vi "Driving Simulator.vi"() -> ()   [LabVIEW 2019]
uses:
  <vilib>/Utility/NIReport.llb/Report Type.ctl
  <vilib>/Instr/_visa.llb/VISA Configure Serial Port (Instr).vi
  <vilib>/Utility/inputDevices.llb/joystickAcquire.vi
  <vilib>/addons/_office/excel.llb/Excel Easy Table (num).vi
  <vilib>/Utility/NIReport.llb/NI_report.lvclass
  <vilib>/addons/_office/NI_ReportGenerationToolkit.lvlib
  <vilib>/Utility/NIReport.llb/NI_ReportGenerationCore.lvlib
panel:
  out "BRdisp 3":i32(slide) caption="Brake" scale=0.0..100.0
  out "revStateTest 2":bool caption="Reverse"
  out "hbStateTest 2":bool caption="Hand Brake"
  out "THdisp 2":i32(slide) caption="Throtle" scale=0.0..100.0
  out "SWdisp 2":i32(knob) caption="Steering wheel" scale=0.0..200.0
  out "mPos":cluster{dbl, dbl, dbl}(graph) caption="Motor Positions"
  out "platDisWF":dbl(graph) caption="Displacement"
  out "platPosWF":cluster{"Pitch":dbl, "Roll":dbl, "yaw ":dbl}(graph) caption="Rotations"
  in  "rev":bool caption="reversa"
  in  "hb":bool caption="freno de mano"
  in  "st":i32(knob)=100 caption="volante" scale=0.0..200.0
  in  "br":i32(knob) caption="freno" scale=0.0..100.0
  in  "tr":i32(knob) caption="acelerador" scale=0.0..100.0
  in  "Preferences":bool caption="Edit Simulation Preferences"
  in  "Tab Control 2":enum32{"Input Devices", "IMU", "MCA"}(tab)
  in  "inSel":T1(ring) caption="Select Input Source"
  in  "dispWaveform":bool caption="Display IMU signals?"
  in  "filter":bool=TRUE caption="Filter IMU signals?"
  in  "pitchLIM":dbl=10.0 caption="Pitch Limit"
  in  "xlp":dbl(slide)=0.5 caption="Pitch \nAcceleration \nGain" scale=0.0..0.9 scale format="%#_4g"
  in  "dispMCA":bool caption="Display MCA Output?"
  in  "xhp":dbl(slide)=0.002 caption="Pitch\nVelocity\nGain" scale=0.0..0.02 scale format="%#_4g"
  in  "ylp":dbl(slide)=0.1 caption="Roll\nAcceleration\nGain" scale=0.0..0.2 scale format="%#_4g"
  in  "yhp":dbl(slide)=0.001 caption="Roll\nVelocity\nGain" scale=0.0..0.01 scale format="%#_4g"
  in  "zhp":dbl(slide)=0.02 caption="Heave\nGain" scale=0.0..0.1 scale format="%#_4g"
  in  "rollLIM":dbl=10.0 caption="Roll Limit"
  in  "heaveLIM":dbl=0.01 caption="Heave Limit"
  out "speed":dbl(knob) caption="Speedometer" scale=0.0..100.0
  out "vel":cluster{"vx":dbl, "vy":dbl, "vy":dbl}(graph) caption="Velocity"
  out "acc":cluster{"vx":dbl, "vy":dbl, "vy":dbl}(graph) caption="Acceleration"
  in  "StopSim":bool caption="Stop Simulation"
  out "errorS1":string caption="ERROR Log"
  out "timer":i32(slide) caption="Wating for CARLA to open" scale=0.0..40.0
  in  "sysConf":bool caption="System Configuration"
  in  "Tab Control":T2(tab)
  out "hbStateTest":bool caption="Hand Brake"
  out "revStateTest":bool caption="Reverse"
  out "THdisp":i32(slide) caption="Throtle" scale=0.0..100.0
  in  "startMconf":bool caption="Set Motor Position Manually"
  in  "set":bool caption="Set Current Position as Home"
  in  "m3":i32=90 caption="Motor 3"
  in  "m2":i32=90 caption="Motor 2"
  in  "m1":i32=90 caption="Motor 1"
  in  "extInputsON":bool caption="Imput Devices Connected?"
  in  "controlON":bool caption="Platform Conected?"
  in  "baudRate":i32=115200 caption="Controller Baud Rate"
  in  "XboxON":bool caption="Xbox Controller Connected?"
  in  "TCP Port":i32=10000 caption="CARLA Server TCP Port"
  in  "VISAportC":refnum<visa-resource-name> caption="Controller Serial Port"
  in  "IDbaudRate":i32=115200 caption="Input Devices Baud Rate"
  in  "VISAportID":refnum<visa-resource-name> caption="Input Devices Port"
  out "SWdisp":i32(knob) caption="Steering wheel" scale=0.0..200.0
  out "BRdisp 2":i32(slide) caption="Brake" scale=0.0..100.0
  in  "startIDtest":bool caption="Test Input Devices"
  in  "finishIDtest":bool caption="Finish Testing"
  in  "b":dbl=0.0887 caption="Leg Length"
  in  "a":dbl=0.03 caption="Crank Length"
  in  "z":dbl=0.0887 caption="Platform Height"
  in  "R":dbl=0.0851 caption="Base Radius"
  in  "r":dbl=0.115 caption="Platform Radius"
  in  "record":bool caption="Activate Variable Recording"
  in  "report type":T3=enum."Excel"
  in  "CARLAstat":bool caption="Is CARLA Server Already Running?"
  in  "CARLA Client":path=path "C:/CARLA/PythonAPI/examples/manual_control.py"
  in  "CARLA Server":path=path "C:/CARLA/CarlaUE4.exe"
  in  "Finish":bool caption="Start Simulation"
  out "Status":string caption="Program Status"
  # "* All Dimentions are in meters"
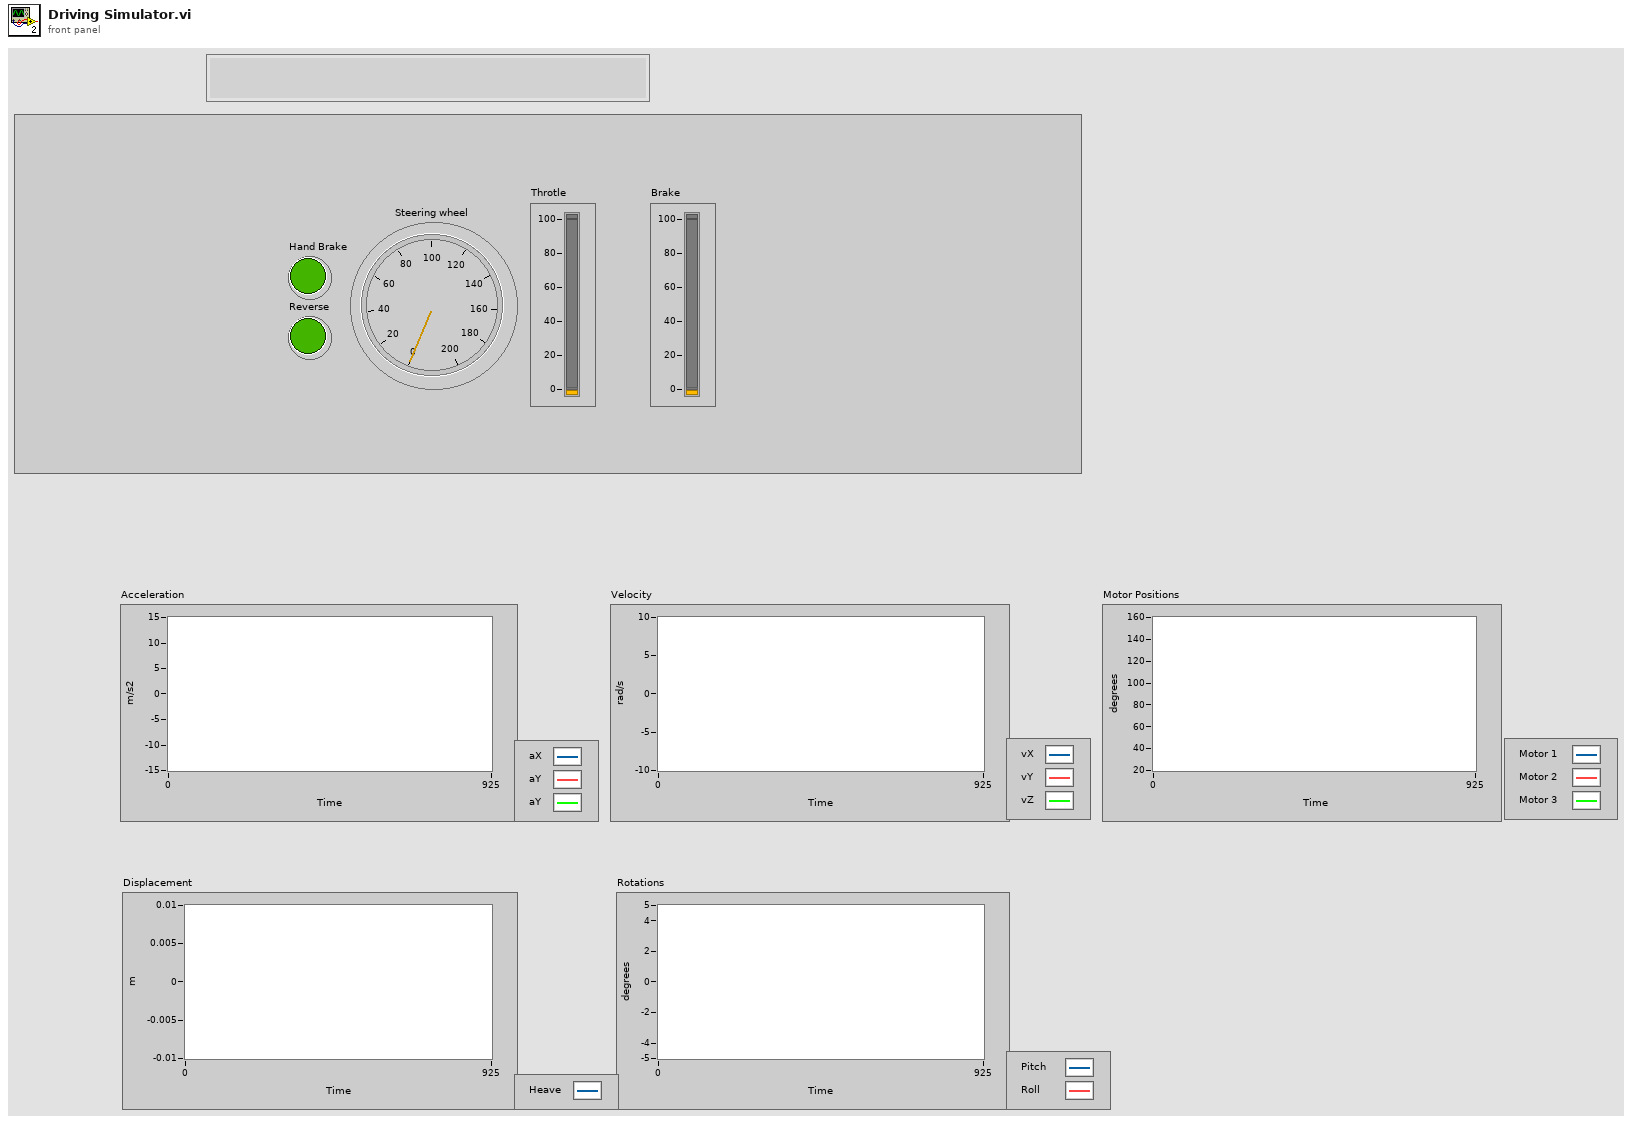
[diagram p1: front panel]
types:
  T1 = enum16{"LabVIEW", "External Devices", "Xbox Controller"}
  T2 = enum32{"Communication", "Platform Dimensions", "Result Recording"}
  T3 = typedef "NI_ReportGenerationCore.lvlib/Report Type.ctl" = enum16{"HTML", "Word", "Excel"}
  T4 = enum8{"Enabled", "Disabled", "Disabled and Grayed Out"}
  T5 = cluster{"st":i32, "tr":i32, "br":i32, "rev":bool, "hb":bool}
  T6 = cluster{"st":i32, "tr":i32, "tr":i32, "hb":bool, "hb":bool}
  T7 = cluster{i32, "Throtle":i32, "Brake":i32, "Reverse":bool, "hand Brake":bool}
  T8 = cluster{"st":i32, "br":i32, "tr":i32, "hb":bool, "rev":bool}
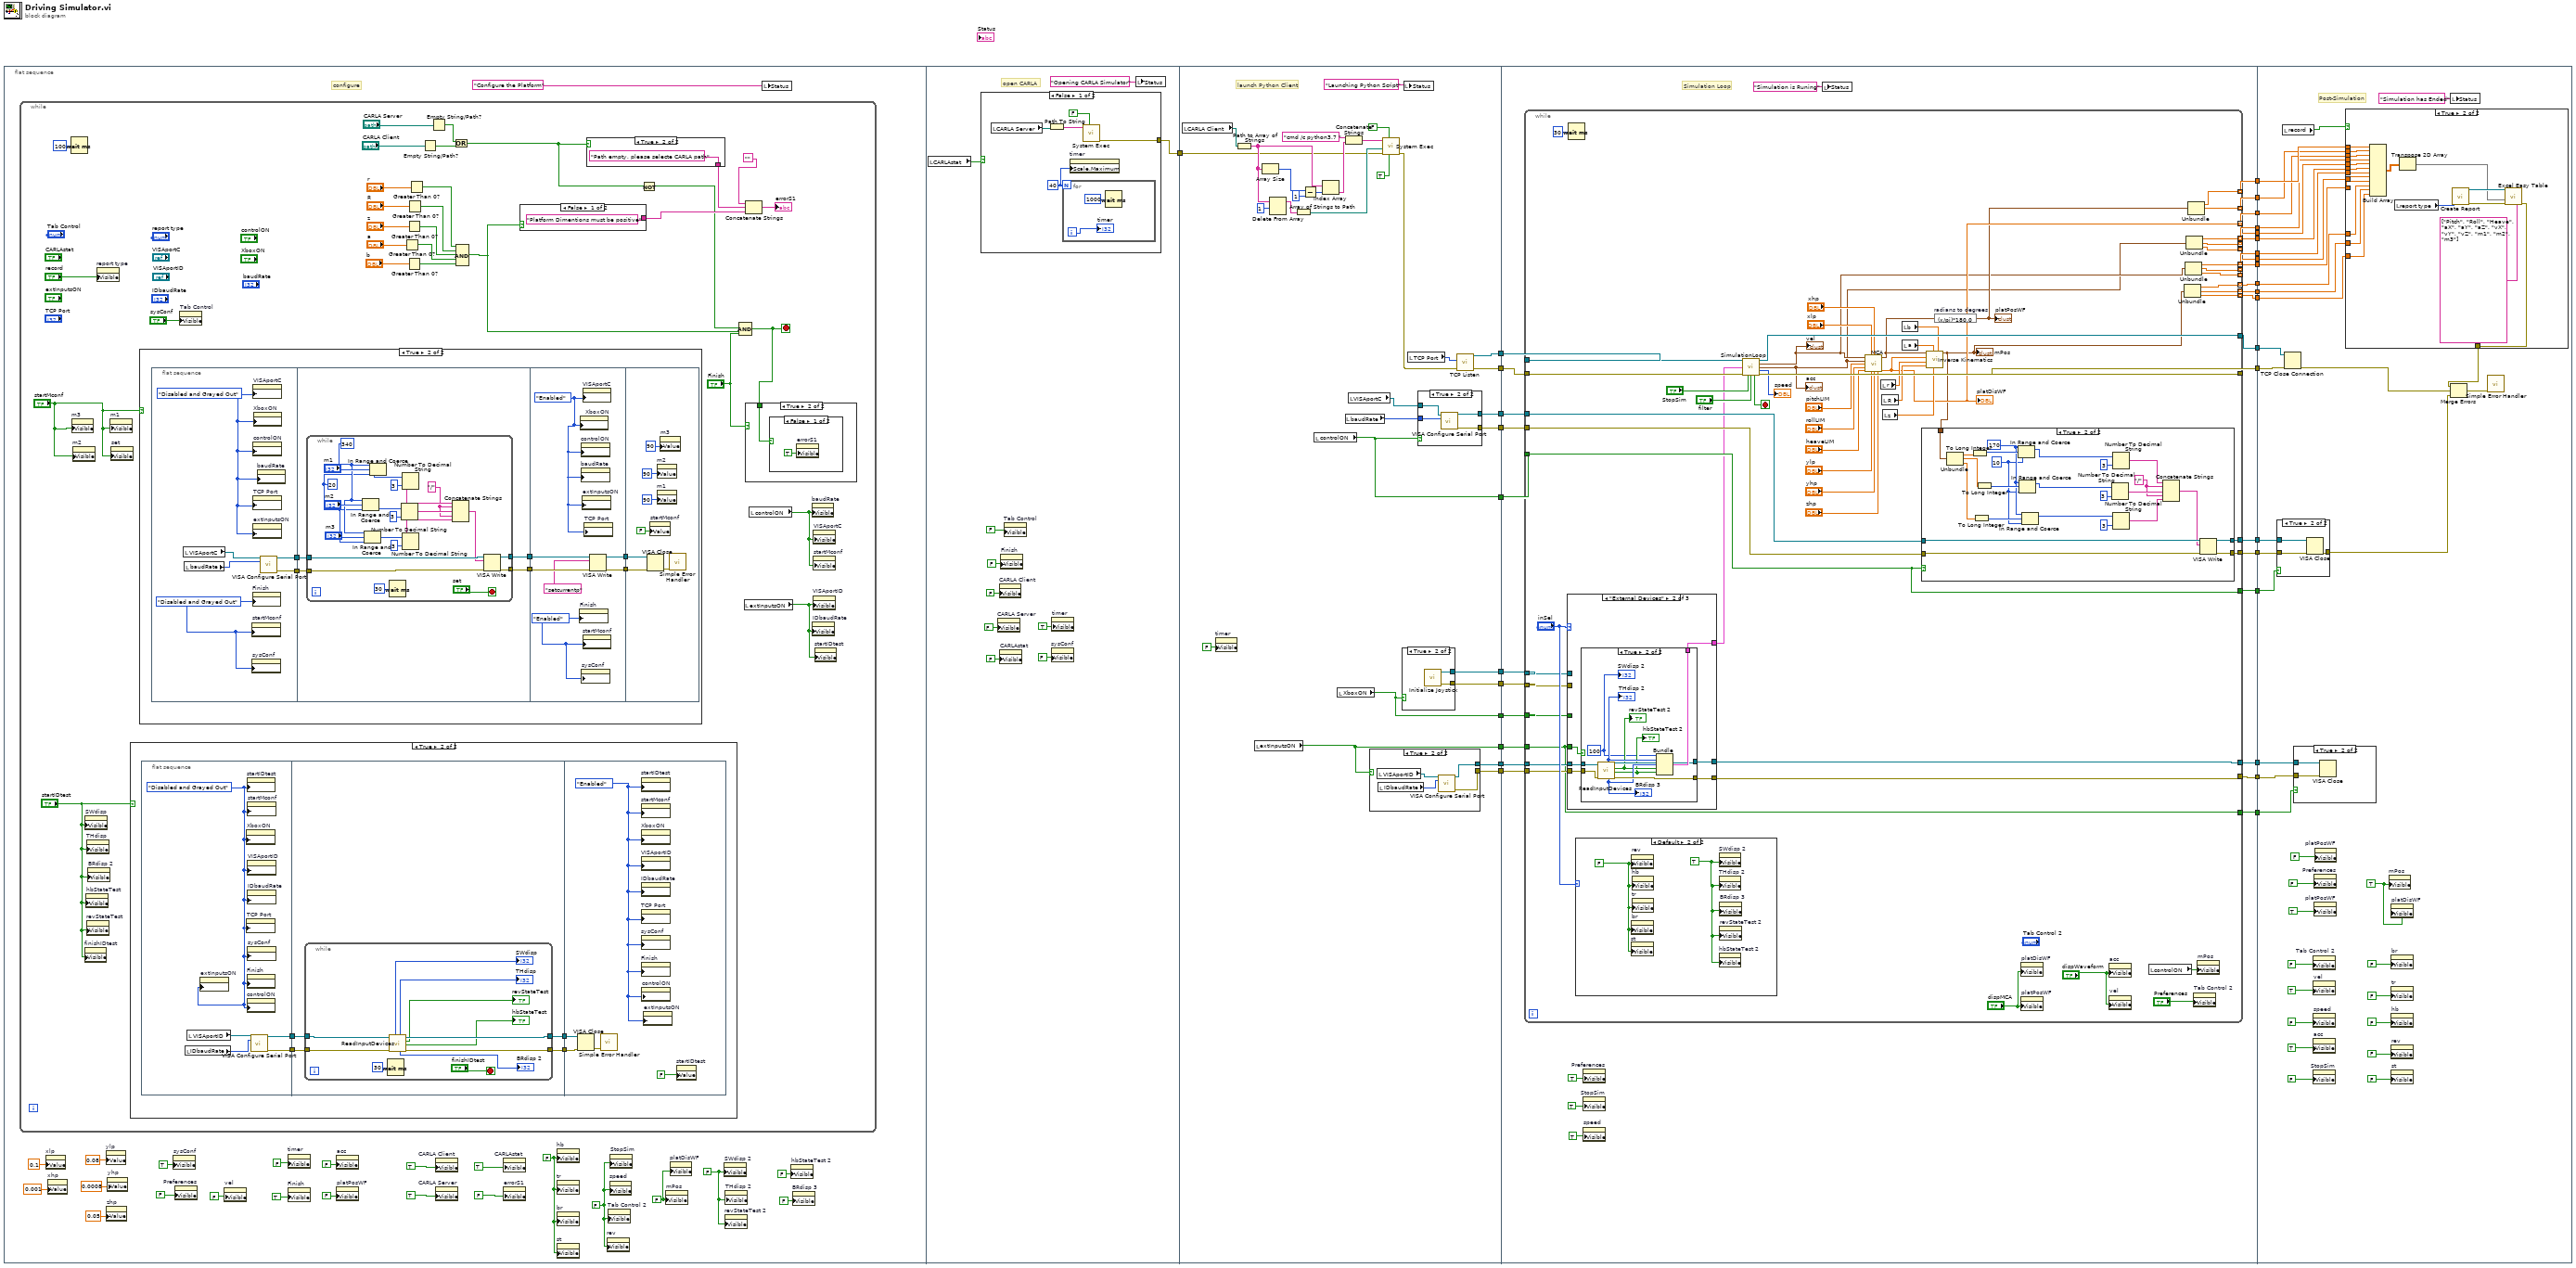
[diagram p0: block diagram]
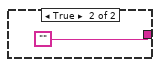
[diagram p4: hidden frame]
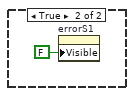
[diagram p6: hidden frame]
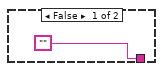
[diagram p7: hidden frame]
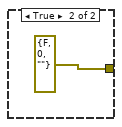
[diagram p8: hidden frame]
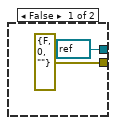
[diagram p9: hidden frame]
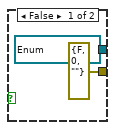
[diagram p10: hidden frame]
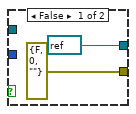
[diagram p11: hidden frame]
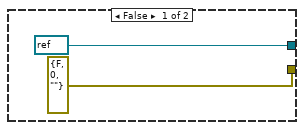
[diagram p12: hidden frame]
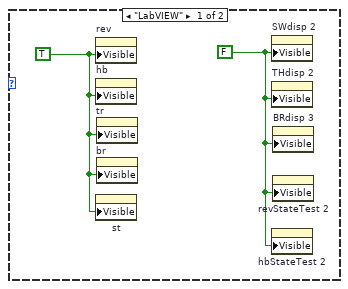
[diagram p13: hidden frame]
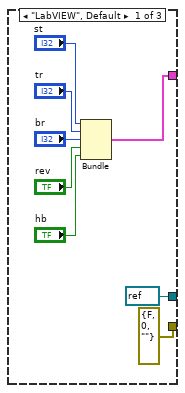
[diagram p14: hidden frame]
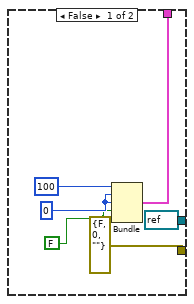
[diagram p15: hidden frame]
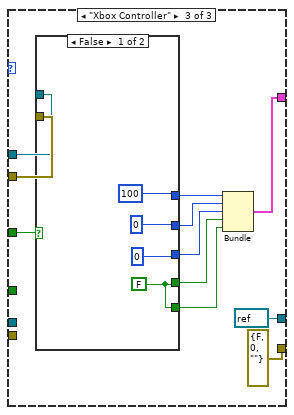
[diagram p16: hidden frame]
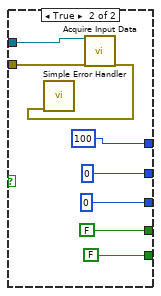
[diagram p17: hidden frame]
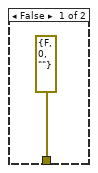
[diagram p19: hidden frame]
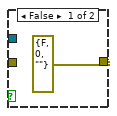
[diagram p20: hidden frame]
diagram:
  n1 = flat-sequence {
    tunnel: [w181] -> w32
    tunnel: w32 -> [w210]
    tunnel: [w208] -> w31
    tunnel: [w207] -> w30
    tunnel: [w205] -> w29
    tunnel: [w204] -> w28
    tunnel: [w199] -> w27
    tunnel: [w202] -> w26
    tunnel: [w201] -> w25
    tunnel: [w200] -> w24
    tunnel: [w194] -> w9
    tunnel: [w193] -> w8
    tunnel: [w192] -> w7
    tunnel: w31 -> [w272]
    tunnel: w30 -> [w271]
    tunnel: [w268] -> w23
    tunnel: [w266] -> w22
    tunnel: w29 -> [w265]
    tunnel: w28 -> [w264]
    tunnel: [w263] -> w21
    tunnel: [w262] -> w20
    tunnel: w27 -> [w261]
    tunnel: [w260] -> w19
    tunnel: w26 -> [w259]
    tunnel: w25 -> [w258]
    tunnel: w24 -> [w257]
    tunnel: [w256] -> w18
    tunnel: [w255] -> w17
    tunnel: [w254] -> w16
    tunnel: [w253] -> w15
    tunnel: [w252] -> w14
    tunnel: [w251] -> w13
    tunnel: [w250] -> w12
    tunnel: [w249] -> w11
    tunnel: [w248] -> w10
    tunnel: w9 -> [w247]
    tunnel: w8 -> [w246]
    tunnel: w7 -> [w245]
    tunnel: [w244] -> w6
    tunnel: [w243] -> w5
    tunnel: [w242] -> w4
    tunnel: [w240] -> w3
    tunnel: [w241] -> w2
    tunnel: [w239] -> w1
    tunnel: w23 -> [w453]
    tunnel: w22 -> [w421]
    tunnel: w21 -> [w439]
    tunnel: w20 -> [w438]
    tunnel: w19 -> [w422]
    tunnel: w18 -> [w436]
    tunnel: w17 -> [w435]
    tunnel: w16 -> [w434]
    tunnel: w15 -> [w433]
    tunnel: w14 -> [w432]
    tunnel: w13 -> [w431]
    tunnel: w12 -> [w430]
    tunnel: w11 -> [w429]
    tunnel: w10 -> [w428]
    tunnel: w6 -> [w420]
    tunnel: w5 -> [w419]
    tunnel: w4 -> [w418]
    tunnel: w3 -> [w416]
    tunnel: w2 -> [w415]
    tunnel: w1 -> [w417]
    frame #0 {
      w35 = FALSE ("Visible")
      w36 = FALSE ("Visible")
      w37 = FALSE ("Visible")
      w38 = FALSE ("Visible")
      # "configure"
      n2 = while {
        stop <- w79 stop-if-true
        n3 = Wait (ms)(milliseconds to wait=u32 100) -> ()  [unwired: 1 out]
        n4 = property on="m3" class="DigNum (strict)"("Visible"="startMconf") -> ()  [unwired: 2 in, 2 out]
        n5 = property on="m2" class="DigNum (strict)"("Visible"="startMconf") -> ()  [unwired: 2 in, 2 out]
        n6 = property on="finishIDtest" class="Bool"("Visible"="startIDtest") -> ()  [unwired: 2 in, 2 out]
        n7 = property on="SWdisp" class="Knob (strict)"("Visible"="startIDtest") -> ()  [unwired: 2 in, 2 out]
        n8 = property on="hbStateTest" class="Bool (strict)"("Visible"="startIDtest") -> ()  [unwired: 2 in, 2 out]
        n9 = property on="THdisp" class="Slide (strict)"("Visible"="startIDtest") -> ()  [unwired: 2 in, 2 out]
        n10 = property on="revStateTest" class="Bool (strict)"("Visible"="startIDtest") -> ()  [unwired: 2 in, 2 out]
        n11 = property on="BRdisp 2" class="Slide (strict)"("Visible"="startIDtest") -> ()  [unwired: 2 in, 2 out]
        n12 = property on="report type" class="Enum (strict)"("Visible"="record") -> ()  [unwired: 2 in, 2 out]
        n13 = property on="m1" class="DigNum (strict)"("Visible"="startMconf") -> ()  [unwired: 2 in, 2 out]
        n14 = property on="set" class="Bool"("Visible"="startMconf") -> ()  [unwired: 2 in, 2 out]
        n15 = case shown="True" "startIDtest" {
          frame False {
          }
          frame True {
            n16 = flat-sequence {
              tunnel: [w94] -> w89
              tunnel: [w93] -> w88
              tunnel: w89 -> [w97]
              tunnel: w88 -> [w98]
              tunnel: [w96] -> w87
              tunnel: [w95] -> w86
              tunnel: w87 -> [w112]
              tunnel: w86 -> [w111]
              frame #0 {
                w90 = T4."Disabled and Grayed Out" ("Disabled")
                n17 = local read "IDbaudRate"() -> (w91:i32)
                n18 = local read "VISAportID"() -> (w92:refnum<visa-resource-name>)
                n19 = property on="extInputsON" class="Bool (strict)"("DisabledEnum"=w90) -> ()  [unwired: 2 in, 2 out]
                n20 = property on="XboxON" class="Bool (strict)"("DisabledEnum"=w90) -> ()  [unwired: 2 in, 2 out]
                n21 = property on="TCP Port" class="DigNum (strict)"("DisabledEnum"=w90) -> ()  [unwired: 2 in, 2 out]
                n22 = property on="startIDtest" class="Bool (strict)"("DisabledEnum"=w90) -> ()  [unwired: 2 in, 2 out]
                n23 = property on="Finish" class="Bool"("DisabledEnum"=w90) -> ()  [unwired: 2 in, 2 out]
                n24 = property on="controlON" class="Bool (strict)"("DisabledEnum"=w90) -> ()  [unwired: 2 in, 2 out]
                n25 = property on="startMconf" class="Bool (strict)"("DisabledEnum"=w90) -> ()  [unwired: 2 in, 2 out]
                n26 = property on="VISAportID" class="VISAName"("DisabledEnum"=w90) -> ()  [unwired: 2 in, 2 out]
                n27 = property on="IDbaudRate" class="DigNum (strict)"("DisabledEnum"=w90) -> ()  [unwired: 2 in, 2 out]
                n28 = property on="sysConf" class="Bool (strict)"("DisabledEnum"=w90) -> ()  [unwired: 2 in, 2 out]
                n29 = call-poly "VISA Configure Serial Port"("VISA resource name"=w92, "baud rate (9600)"=w91) -> ("VISA resource name out"=w94:refnum<visa-resource-name>, "error out"=w93:errorcluster)  [unwired: 12 in]
              }
              frame #1 {
                n30 = while {
                  tunnel: w98 -> [w106]
                  tunnel: w97 -> [w107]
                  tunnel: [w105] -> w96
                  tunnel: [w104] -> w95
                  stop <- "finishIDtest" stop-if-true
                  n31 = Wait (ms)(milliseconds to wait=u32 30) -> ()  [unwired: 1 out]
                  n32 = call "ReadInputDevices.vi"("error in (no error)"=w106, "VISA Refnum in"=w107) -> ("error out"=w104:errorcluster, "hand Brake"=→"hbStateTest":bool, "Reverse"=→"revStateTest":bool, "VISA Refnum out"=w105:refnum<visa-resource-name>, "Brake"=→"BRdisp 2":i32, "Throtle"=→"THdisp":i32, "Steering Wheel"=→"SWdisp":i32)  [unwired: 3 in]
                }
              }
              frame #2 {
                w110 = T4."Enabled" ("Disabled")
                n33 = VISA Close(VISA resource name=w112, error in (no error)=w111) -> (error out=w114:errorcluster)
                n34 = call <vilib>:"Simple Error Handler.vi"("error in (no error)"=w114) -> ()  [unwired: 4 in, 5 out]
                n35 = property on="startIDtest" class="Bool (strict)"("DisabledEnum"=w110) -> ()  [unwired: 2 in, 2 out]
                n36 = property on="startMconf" class="Bool (strict)"("DisabledEnum"=w110) -> ()  [unwired: 2 in, 2 out]
                n37 = property on="XboxON" class="Bool (strict)"("DisabledEnum"=w110) -> ()  [unwired: 2 in, 2 out]
                n38 = property on="VISAportID" class="VISAName"("DisabledEnum"=w110) -> ()  [unwired: 2 in, 2 out]
                n39 = property on="IDbaudRate" class="DigNum (strict)"("DisabledEnum"=w110) -> ()  [unwired: 2 in, 2 out]
                n40 = property on="TCP Port" class="DigNum (strict)"("DisabledEnum"=w110) -> ()  [unwired: 2 in, 2 out]
                n41 = property on="sysConf" class="Bool (strict)"("DisabledEnum"=w110) -> ()  [unwired: 2 in, 2 out]
                n42 = property on="Finish" class="Bool"("DisabledEnum"=w110) -> ()  [unwired: 2 in, 2 out]
                n43 = property on="controlON" class="Bool (strict)"("DisabledEnum"=w110) -> ()  [unwired: 2 in, 2 out]
                n44 = property on="extInputsON" class="Bool (strict)"("DisabledEnum"=w110) -> ()  [unwired: 2 in, 2 out]
                n45 = property on="startIDtest" class="Bool (strict)"("Value"=FALSE ("startMconf")) -> ()  [unwired: 2 in, 2 out]
              }
            }
          }
        }
        n46 = case shown="True" "startMconf" {
          frame False {
          }
          frame True {
            n47 = flat-sequence {
              tunnel: [w124] -> w120
              tunnel: [w123] -> w119
              tunnel: w120 -> [w129]
              tunnel: w119 -> [w130]
              tunnel: [w128] -> w118
              tunnel: [w127] -> w117
              tunnel: w118 -> [w159]
              tunnel: w117 -> [w158]
              tunnel: [w156] -> w116
              tunnel: [w155] -> w115
              tunnel: w116 -> [w166]
              tunnel: w115 -> [w165]
              frame #0 {
                w122 = T4."Disabled and Grayed Out" ("Disabled")
                w121 = T4."Disabled and Grayed Out" ("Disabled")
                n48 = local read "VISAportC"() -> (w126:refnum<visa-resource-name>)
                n49 = local read "baudRate"() -> (w125:i32)
                n50 = property on="startMconf" class="Bool (strict)"("DisabledEnum"=w122) -> ()  [unwired: 2 in, 2 out]
                n51 = property on="sysConf" class="Bool (strict)"("DisabledEnum"=w122) -> ()  [unwired: 2 in, 2 out]
                n52 = property on="Finish" class="Bool"("DisabledEnum"=w122) -> ()  [unwired: 2 in, 2 out]
                n53 = property on="VISAportC" class="VISAName"("DisabledEnum"=w121) -> ()  [unwired: 2 in, 2 out]
                n54 = property on="controlON" class="Bool (strict)"("DisabledEnum"=w121) -> ()  [unwired: 2 in, 2 out]
                n55 = property on="TCP Port" class="DigNum (strict)"("DisabledEnum"=w121) -> ()  [unwired: 2 in, 2 out]
                n56 = property on="extInputsON" class="Bool (strict)"("DisabledEnum"=w121) -> ()  [unwired: 2 in, 2 out]
                n57 = property on="XboxON" class="Bool (strict)"("DisabledEnum"=w121) -> ()  [unwired: 2 in, 2 out]
                n58 = property on="baudRate" class="DigNum (strict)"("DisabledEnum"=w121) -> ()  [unwired: 2 in, 2 out]
                n59 = call-poly "VISA Configure Serial Port"("VISA resource name"=w126, "baud rate (9600)"=w125) -> ("VISA resource name out"=w124:refnum<visa-resource-name>, "error out"=w123:errorcluster)  [unwired: 12 in]
              }
              frame #1 {
                n60 = while {
                  tunnel: w130 -> [w152]
                  tunnel: w129 -> [w151]
                  tunnel: [w134] -> w128
                  tunnel: [w133] -> w127
                  stop <- "set" stop-if-true
                  w135 = 20 ("lower limit")
                  w136 = 340 ("upper limit")
                  w144 = "/"
                  n61 = In Range and Coerce(upper limit=w136, x="m2", lower limit=w135) -> (coerced(x)=w138:i32)  [unwired: 1 out]
                  n62 = In Range and Coerce(upper limit=w136, x="m3", lower limit=w135) -> (coerced(x)=w137:i32)  [unwired: 1 out]
                  n63 = In Range and Coerce(upper limit=w136, x="m1", lower limit=w135) -> (coerced(x)=w141:i32)  [unwired: 1 out]
                  n64 = Wait (ms)(milliseconds to wait=u32 30) -> ()  [unwired: 1 out]
                  n65 = Number To Decimal String(number=w138, width (-)=i16 3) -> (decimal integer string=w149:string)
                  n66 = Number To Decimal String(number=w141, width (-)=i16 3) -> (decimal integer string=w148:string)
                  n67 = Number To Decimal String(number=w137, width (-)=i16 3) -> (decimal integer string=w150:string)
                  n68 = Concatenate Strings(w148, w144, w149, w144, w150) -> (w143:string)
                  n69 = VISA Write(VISA resource name=w151, write buffer=w143, error in (no error)=w152) -> (VISA resource name out=w134:refnum<visa-resource-name>, error out=w133:errorcluster)  [unwired: 1 out]
                }
              }
              frame #2 {
                w153 = T4."Enabled" ("Disabled")
                w154 = T4."Enabled" ("Disabled")
                n70 = property on="Finish" class="Bool"("DisabledEnum"=w153) -> ()  [unwired: 2 in, 2 out]
                n71 = property on="XboxON" class="Bool (strict)"("DisabledEnum"=w154) -> ()  [unwired: 2 in, 2 out]
                n72 = property on="controlON" class="Bool (strict)"("DisabledEnum"=w154) -> ()  [unwired: 2 in, 2 out]
                n73 = property on="baudRate" class="DigNum (strict)"("DisabledEnum"=w154) -> ()  [unwired: 2 in, 2 out]
                n74 = property on="sysConf" class="Bool (strict)"("DisabledEnum"=w153) -> ()  [unwired: 2 in, 2 out]
                n75 = property on="extInputsON" class="Bool (strict)"("DisabledEnum"=w154) -> ()  [unwired: 2 in, 2 out]
                n76 = property on="VISAportC" class="VISAName"("DisabledEnum"=w154) -> ()  [unwired: 2 in, 2 out]
                n77 = property on="startMconf" class="Bool (strict)"("DisabledEnum"=w153) -> ()  [unwired: 2 in, 2 out]
                n78 = property on="TCP Port" class="DigNum (strict)"("DisabledEnum"=w154) -> ()  [unwired: 2 in, 2 out]
                n79 = VISA Write(VISA resource name=w159, write buffer="setcurrentp", error in (no error)=w158) -> (VISA resource name out=w156:refnum<visa-resource-name>, error out=w155:errorcluster)  [unwired: 1 out]
              }
              frame #3 {
                n80 = VISA Close(VISA resource name=w166, error in (no error)=w165) -> (error out=w164:errorcluster)
                n81 = property on="startMconf" class="Bool (strict)"("Value"=FALSE ("startMconf")) -> ()  [unwired: 2 in, 2 out]
                n82 = property on="m2" class="DigNum (strict)"("Value"=90 ("m2")) -> ()  [unwired: 2 in, 2 out]
                n83 = property on="m1" class="DigNum (strict)"("Value"=90 ("m1")) -> ()  [unwired: 2 in, 2 out]
                n84 = property on="m3" class="DigNum (strict)"("Value"=90 ("m3")) -> ()  [unwired: 2 in, 2 out]
                n85 = call <vilib>:"Simple Error Handler.vi"("error in (no error)"=w164) -> ()  [unwired: 4 in, 5 out]
              }
            }
          }
        }
        n86 = property on="Tab Control" class="TabCtl (strict)"("Visible"="sysConf") -> ()  [unwired: 2 in, 2 out]
        n87 = Greater Than 0?(x="a") -> (x > 0?=w73:bool)
        n88 = Greater Than 0?(x="z") -> (x > 0?=w74:bool)
        n89 = Greater Than 0?(x="b") -> (x > 0?=w72:bool)
        n90 = Greater Than 0?(x="R") -> (x > 0?=w75:bool)
        n91 = Greater Than 0?(x="r") -> (x > 0?=w76:bool)
        n92 = Empty String/Path?(string/path="CARLA Client") -> (empty?=w78:bool)
        n93 = Empty String/Path?(string/path="CARLA Server") -> (empty?=w83:bool)
        n94 = Or(x=w83, y=w78) -> (x .or. y?=w68:bool)
        n95 = Compound Arithmetic op=AND(w76, w75, w74, w73, w72) -> (w69:bool)
        n96 = case shown="False" w69 {
          tunnel: ["Platform Dimentions must be positive" ""] -> w71
          frame False {
          }
          frame True {
          }
        }
        n97 = case shown="True" w68 {
          tunnel: ["" "Path empty, please selecte CARLA path" ("string")] -> w81
          frame False {
          }
          frame True {
          }
        }
        n98 = Not(x=w68) -> (.not. x?=w67:bool)
        n99 = Compound Arithmetic op=AND(w67, w69, "Finish") -> (w79:bool)
        n100 = local read "extInputsON"() -> (w56:bool)
        n101 = Concatenate Strings("", w81, w71) -> (→"errorS1":string)
        n102 = case shown="True" "Finish" {
          tunnel: w79 -> [_ w169]
          frame False {
          }
          frame True {
            n103 = case shown="False" w169 {
              frame False {
                n104 = property on="errorS1" class="Str"("Visible"=TRUE) -> ()  [unwired: 2 in, 2 out]
              }
              frame True {
                n105 = property on="errorS1" class="Str"("Visible"=FALSE) -> ()  [unwired: 2 in, 2 out]
              }
            }
          }
        }
        n106 = local read "controlON"() -> (w59:bool)
        n107 = property on="baudRate" class="DigNum (strict)"("Visible"=w59) -> ()  [unwired: 2 in, 2 out]
        n108 = property on="IDbaudRate" class="DigNum (strict)"("Visible"=w56) -> ()  [unwired: 2 in, 2 out]
        n109 = property on="VISAportID" class="VISAName"("Visible"=w56) -> ()  [unwired: 2 in, 2 out]
        n110 = property on="VISAportC" class="VISAName"("Visible"=w59) -> ()  [unwired: 2 in, 2 out]
        n111 = property on="startMconf" class="Bool (strict)"("Visible"=w59) -> ()  [unwired: 2 in, 2 out]
        n112 = property on="startIDtest" class="Bool (strict)"("Visible"=w56) -> ()  [unwired: 2 in, 2 out]
      }
      n113 = property on="xlp" class="Slide (strict)"("Value"=0.1 ("xlp")) -> ()  [unwired: 2 in, 2 out]
      n114 = property on="xhp" class="Slide (strict)"("Value"=0.001 ("xhp")) -> ()  [unwired: 2 in, 2 out]
      n115 = property on="ylp" class="Slide (strict)"("Value"=0.08 ("ylp")) -> ()  [unwired: 2 in, 2 out]
      n116 = property on="zhp" class="Slide (strict)"("Value"=0.05 ("zhp")) -> ()  [unwired: 2 in, 2 out]
      n117 = property on="yhp" class="Slide (strict)"("Value"=0.0008 ("yhp")) -> ()  [unwired: 2 in, 2 out]
      n118 = property on="sysConf" class="Bool (strict)"("Visible"=TRUE) -> ()  [unwired: 2 in, 2 out]
      n119 = property on="Preferences" class="Bool (strict)"("Visible"=FALSE) -> ()  [unwired: 2 in, 2 out]
      n120 = property on="vel" class="WFChart (strict)"("Visible"=FALSE) -> ()  [unwired: 2 in, 2 out]
      n121 = property on="timer" class="Slide (strict)"("Visible"=FALSE) -> ()  [unwired: 2 in, 2 out]
      n122 = property on="Finish" class="Bool"("Visible"=TRUE) -> ()  [unwired: 2 in, 2 out]
      n123 = property on="acc" class="WFChart (strict)"("Visible"=FALSE) -> ()  [unwired: 2 in, 2 out]
      n124 = property on="platPosWF" class="WFChart (strict)"("Visible"=FALSE) -> ()  [unwired: 2 in, 2 out]
      n125 = property on="CARLA Client" class="Path"("Visible"=TRUE) -> ()  [unwired: 2 in, 2 out]
      n126 = property on="CARLA Server" class="Path"("Visible"=TRUE) -> ()  [unwired: 2 in, 2 out]
      n127 = property on="CARLAstat" class="Bool (strict)"("Visible"=TRUE) -> ()  [unwired: 2 in, 2 out]
      n128 = property on="errorS1" class="Str"("Visible"=FALSE) -> ()  [unwired: 2 in, 2 out]
      n129 = property on="hb" class="Bool (strict)"("Visible"=w38) -> ()  [unwired: 2 in, 2 out]
      n130 = property on="tr" class="Knob (strict)"("Visible"=w38) -> ()  [unwired: 2 in, 2 out]
      n131 = property on="br" class="Knob (strict)"("Visible"=w38) -> ()  [unwired: 2 in, 2 out]
      n132 = property on="st" class="Knob (strict)"("Visible"=w38) -> ()  [unwired: 2 in, 2 out]
      n133 = property on="rev" class="Bool (strict)"("Visible"=w37) -> ()  [unwired: 2 in, 2 out]
      n134 = property on="Tab Control 2" class="TabCtl (strict)"("Visible"=w37) -> ()  [unwired: 2 in, 2 out]
      n135 = property on="speed" class="Knob (strict)"("Visible"=w37) -> ()  [unwired: 2 in, 2 out]
      n136 = property on="StopSim" class="Bool"("Visible"=w37) -> ()  [unwired: 2 in, 2 out]
      n137 = property on="mPos" class="WFChart (strict)"("Visible"=w36) -> ()  [unwired: 2 in, 2 out]
      n138 = property on="platDisWF" class="WFChart (strict)"("Visible"=w36) -> ()  [unwired: 2 in, 2 out]
      n139 = property on="SWdisp 2" class="Knob (strict)"("Visible"=w35) -> ()  [unwired: 2 in, 2 out]
      n140 = property on="revStateTest 2" class="Bool (strict)"("Visible"=w35) -> ()  [unwired: 2 in, 2 out]
      n141 = property on="THdisp 2" class="Slide (strict)"("Visible"=w35) -> ()  [unwired: 2 in, 2 out]
      n142 = local write "Status"("Configure the Platform" ("String")) -> ()
      n143 = property on="hbStateTest 2" class="Bool (strict)"("Visible"=FALSE) -> ()  [unwired: 2 in, 2 out]
      n144 = property on="BRdisp 3" class="Slide (strict)"("Visible"=FALSE) -> ()  [unwired: 2 in, 2 out]
    }
    frame #1 {
      # "open CARLA"
      n145 = local read "CARLAstat"() -> (w174:bool)
      n146 = case shown="False" w174 {
        tunnel: [w186 errorcluster {"status"=FALSE, "code"=0, "source"=""} ("error out")] -> w181
        frame False {
          w185 = 40
          n147 = local read "CARLA Server"() -> (w184:path)
          n148 = Path To String(path=w184) -> (string=w188:string)
          n149 = for {
            N: w185 -> [_]
            i -> [w190]
            n150 = Wait (ms)(milliseconds to wait=u32 1000) -> ()  [unwired: 1 out]
            "timer" <- w190
          }
          n151 = property on="timer" class="Slide (strict)"("Scale.Maximum"=w185) -> ()  [unwired: 2 in, 2 out]
          n152 = call <vilib>:"System Exec.vi"("wait until completion? (T)"=FALSE, "command line"=w188) -> ("error out"=w186:errorcluster)  [unwired: 6 in, 3 out]
        }
        frame True {
        }
      }
      n153 = property on="CARLA Server" class="Path"("Visible"=FALSE) -> ()  [unwired: 2 in, 2 out]
      n154 = property on="CARLA Client" class="Path"("Visible"=FALSE) -> ()  [unwired: 2 in, 2 out]
      n155 = property on="CARLAstat" class="Bool (strict)"("Visible"=FALSE) -> ()  [unwired: 2 in, 2 out]
      n156 = property on="Finish" class="Bool"("Visible"=FALSE) -> ()  [unwired: 2 in, 2 out]
      n157 = property on="Tab Control" class="TabCtl (strict)"("Visible"=FALSE) -> ()  [unwired: 2 in, 2 out]
      n158 = property on="sysConf" class="Bool (strict)"("Visible"=FALSE) -> ()  [unwired: 2 in, 2 out]
      n159 = property on="timer" class="Slide (strict)"("Visible"=TRUE) -> ()  [unwired: 2 in, 2 out]
      n160 = local write "Status"("Opening CARLA Simulator" ("String")) -> ()
    }
    frame #2 {
      # "launch Python Client"
      n161 = local read "CARLA Client"() -> (w196:path)
      n162 = property on="timer" class="Slide (strict)"("Visible"=FALSE) -> ()  [unwired: 2 in, 2 out]
      n163 = Path to Array of Strings(0:w196) -> (2:w216:string[])  [unwired: 1 out]
      n164 = local read "extInputsON"() -> (w192:bool)
      n165 = Array Size(array=w216) -> (size(s)=w215:i32)
      n166 = Delete From Array(array=w216, length=1) -> (array with subset deleted=w218:string[])  [unwired: 1 in, 1 out]
      n167 = Array of Strings to Path(0:w218) -> (2:w221:path)  [unwired: 1 in]
      n168 = Subtract(x=w215, y=1) -> (x-y=w217:i32)
      n169 = local read "controlON"() -> (w199:bool)
      n170 = Index Array(array=w216, index=w217) -> (element=w220:string)
      n171 = local read "XboxON"() -> (w200:bool)
      n172 = local read "baudRate"() -> (w198:i32)
      n173 = Concatenate Strings("cmd /c python3.7 " ("string"), w220) -> (w219:string)
      n174 = local read "VISAportC"() -> (w195:refnum<visa-resource-name>)
      n175 = case shown="True" w192 {
        tunnel: [refnum<visa-resource-name> refnum ("VISA resource name out") w228] -> w194
        tunnel: [errorcluster {"status"=FALSE, "code"=0, "source"=""} ("error out") w227] -> w193
        frame False {
        }
        frame True {
          n176 = local read "VISAportID"() -> (w225:refnum<visa-resource-name>)
          n177 = local read "IDbaudRate"() -> (w226:i32)
          n178 = call-poly "VISA Configure Serial Port"("VISA resource name"=w225, "baud rate (9600)"=w226) -> ("VISA resource name out"=w228:refnum<visa-resource-name>, "error out"=w227:errorcluster)  [unwired: 12 in]
        }
      }
      n179 = call <vilib>:"System Exec.vi"("run minimized? (F)"=TRUE, "wait until completion? (T)"=FALSE, "error in (no error)"=w210, "working directory"=w221, "command line"=w219) -> ("error out"=w203:errorcluster)  [unwired: 3 in, 3 out]
      n180 = case shown="True" w200 {
        tunnel: [w230 w232] -> w202
        tunnel: [errorcluster {"status"=FALSE, "code"=0, "source"=""} ("error out") w231] -> w201
        frame False {
          w230 = refnum<k1> refnum items=["JOYSTICK"] ("device ID")
        }
        frame True {
          n181 = call <vilib>:"Initialize Joystick.vi"() -> ("error out"=w231:errorcluster, "device ID"=w232:refnum<k1>)  [unwired: 10 in]
        }
      }
      n182 = local write "Status"("Launching Python Script" ("String")) -> ()
      n183 = local read "TCP Port"() -> (w197:i32)
      n184 = case shown="True" w199 {
        tunnel: w198 -> [_ w238]
        tunnel: [refnum<visa-resource-name> refnum ("VISA resource name out") w237] -> w205
        tunnel: [errorcluster {"status"=FALSE, "code"=0, "source"=""} ("error out") w236] -> w204
        tunnel: w195 -> [_ w235]
        frame False {
        }
        frame True {
          n185 = call-poly "VISA Configure Serial Port"("VISA resource name"=w235, "baud rate (9600)"=w238) -> ("VISA resource name out"=w237:refnum<visa-resource-name>, "error out"=w236:errorcluster)  [unwired: 12 in]
        }
      }
      n186 = call <vilib>:"TCP Listen.vi"("error in (no error)"=w203, "port"=w197) -> ("error out"=w207:errorcluster, "connection ID"=w208:refnum<k5>)  [unwired: 5 in, 3 out]
    }
    frame #3 {
      # "Simulation Loop"
      n187 = while {
        tunnel: w272 -> [w331]
        tunnel: [w329] -> w266
        tunnel: w271 -> [w330]
        tunnel: [w328] -> w268
        tunnel: w265 -> [w311]
        tunnel: w264 -> [w312]
        tunnel: [w310] -> w263
        tunnel: [w309] -> w262
        tunnel: w261 -> [w308]
        tunnel: [w308] -> w260
        tunnel: w259 -> [w307]
        tunnel: w258 -> [w306]
        tunnel: w257 -> [w305]
        tunnel: [w296] -> w256 mode=indexing
        tunnel: [w295] -> w255 mode=indexing
        tunnel: [w293] -> w254 mode=indexing
        tunnel: [w292] -> w253 mode=indexing
        tunnel: [w291] -> w252 mode=indexing
        tunnel: [w290] -> w251 mode=indexing
        tunnel: [w289] -> w250 mode=indexing
        tunnel: [w288] -> w249 mode=indexing
        tunnel: [w287] -> w248 mode=indexing
        tunnel: w247 -> [w282]
        tunnel: w246 -> [w281]
        tunnel: w245 -> [w278]
        tunnel: [w280] -> w244
        tunnel: [w279] -> w243
        tunnel: [w278] -> w242
        tunnel: [w276] -> w239 mode=indexing
        tunnel: [w275] -> w240 mode=indexing
        tunnel: [w274] -> w241 mode=indexing
        stop <- w327 stop-if-true
        n188 = case shown="\"External Devices\"" "inSel" {
          tunnel: w307 -> [_ _ w400]
          tunnel: w306 -> [_ _ w401]
          tunnel: w305 -> [_ _ w402]
          tunnel: [w364 w375 w394] -> w283
          tunnel: w282 -> [_ w374 _]
          tunnel: w281 -> [_ w373 _]
          tunnel: w278 -> [_ w372 _]
          tunnel: [refnum<visa-resource-name> refnum ("VISA Refnum out") w371 refnum<visa-resource-name> refnum ("VISA Refnum out")] -> w280
          tunnel: [errorcluster {"status"=FALSE, "code"=0, "source"=""} ("error out") w370 errorcluster {"status"=FALSE, "code"=0, "source"=""} ("error out")] -> w279
          frame "LabVIEW", Default {
            n189 = Bundle("st"="st", "tr"="tr", "br"="br", "rev"="rev", "hb"="hb") -> (w364:T5)  [unwired: 1 in]
          }
          frame "External Devices" {
            n190 = case shown="True" w372 {
              tunnel: [w378 w391] -> w375
              tunnel: w374 -> [_ w390]
              tunnel: w373 -> [_ w389]
              tunnel: [refnum<visa-resource-name> refnum ("VISA Refnum out") w388] -> w371
              tunnel: [errorcluster {"status"=FALSE, "code"=0, "source"=""} ("error out") w387] -> w370
              frame False {
                w379 = FALSE ("hb")
                w380 = 0 ("tr")
                n191 = Bundle("st"=100, "tr"=w380, "tr"=w380, "hb"=w379, "hb"=w379) -> (w378:T6)  [unwired: 1 in]
              }
              frame True {
                w382 = 100
                n192 = call "ReadInputDevices.vi"("error in (no error)"=w389, "VISA Refnum in"=w390) -> ("error out"=w387:errorcluster, "hand Brake"=w383:bool, "Reverse"=w384:bool, "VISA Refnum out"=w388:refnum<visa-resource-name>, "Brake"=w385:i32, "Throtle"=w386:i32)  [unwired: 3 in, 1 out]
                "THdisp 2" <- w386
                "BRdisp 3" <- w385
                "revStateTest 2" <- w384
                "hbStateTest 2" <- w383
                n193 = Bundle(w382, "Throtle"=w386, "Brake"=w385, "Reverse"=w384, "hand Brake"=w383) -> (w391:T7)  [unwired: 1 in]
                "SWdisp 2" <- w382
              }
            }
          }
          frame "Xbox Controller" {
            n194 = case shown="False" w402 {
              tunnel: w400 -> [_ w414]
              tunnel: w401 -> [_ w413]
              tunnel: [100 ("st") 100 ("st")] -> w399
              tunnel: [0 ("tr") 0 ("br")] -> w398
              tunnel: [0 ("br") 0 ("tr")] -> w397
              tunnel: [w403 FALSE ("hb")] -> w396
              tunnel: [w403 FALSE ("rev")] -> w395
              frame False {
                w403 = FALSE ("hb")
              }
              frame True {
                n195 = call-poly <vilib>:"Acquire Input Data.vi"("device ID"=w414, "error in (no error)"=w413) -> ("error out"=w412:errorcluster)  [unwired: 13 in, 4 out]
                n196 = call <vilib>:"Simple Error Handler.vi"("error in (no error)"=w412) -> ()  [unwired: 4 in, 5 out]
              }
            }
            n197 = Bundle("st"=w399, "br"=w398, "tr"=w397, "hb"=w396, "rev"=w395) -> (w394:T8)  [unwired: 1 in]
          }
        }
        n198 = Wait (ms)(milliseconds to wait=u32 30) -> ()  [unwired: 1 out]
        n199 = case shown="Default" "inSel" {
          frame "LabVIEW" {
            w358 = FALSE ("Visible")
            w359 = TRUE ("Visible")
            n200 = property on="rev" class="Bool (strict)"("Visible"=w359) -> ()  [unwired: 2 in, 2 out]
            n201 = property on="hb" class="Bool (strict)"("Visible"=w359) -> ()  [unwired: 2 in, 2 out]
            n202 = property on="st" class="Knob (strict)"("Visible"=w359) -> ()  [unwired: 2 in, 2 out]
            n203 = property on="tr" class="Knob (strict)"("Visible"=w359) -> ()  [unwired: 2 in, 2 out]
            n204 = property on="br" class="Knob (strict)"("Visible"=w359) -> ()  [unwired: 2 in, 2 out]
            n205 = property on="SWdisp 2" class="Knob (strict)"("Visible"=w358) -> ()  [unwired: 2 in, 2 out]
            n206 = property on="THdisp 2" class="Slide (strict)"("Visible"=w358) -> ()  [unwired: 2 in, 2 out]
            n207 = property on="hbStateTest 2" class="Bool (strict)"("Visible"=w358) -> ()  [unwired: 2 in, 2 out]
            n208 = property on="BRdisp 3" class="Slide (strict)"("Visible"=w358) -> ()  [unwired: 2 in, 2 out]
            n209 = property on="revStateTest 2" class="Bool (strict)"("Visible"=w358) -> ()  [unwired: 2 in, 2 out]
          }
          frame Default {
            w360 = TRUE ("Visible")
            w361 = FALSE ("Visible")
            n210 = property on="rev" class="Bool (strict)"("Visible"=w361) -> ()  [unwired: 2 in, 2 out]
            n211 = property on="br" class="Knob (strict)"("Visible"=w361) -> ()  [unwired: 2 in, 2 out]
            n212 = property on="st" class="Knob (strict)"("Visible"=w361) -> ()  [unwired: 2 in, 2 out]
            n213 = property on="hb" class="Bool (strict)"("Visible"=w361) -> ()  [unwired: 2 in, 2 out]
            n214 = property on="tr" class="Knob (strict)"("Visible"=w361) -> ()  [unwired: 2 in, 2 out]
            n215 = property on="SWdisp 2" class="Knob (strict)"("Visible"=w360) -> ()  [unwired: 2 in, 2 out]
            n216 = property on="THdisp 2" class="Slide (strict)"("Visible"=w360) -> ()  [unwired: 2 in, 2 out]
            n217 = property on="hbStateTest 2" class="Bool (strict)"("Visible"=w360) -> ()  [unwired: 2 in, 2 out]
            n218 = property on="BRdisp 3" class="Slide (strict)"("Visible"=w360) -> ()  [unwired: 2 in, 2 out]
            n219 = property on="revStateTest 2" class="Bool (strict)"("Visible"=w360) -> ()  [unwired: 2 in, 2 out]
          }
        }
        n220 = call "SimulationLoop.vi"("connection ID"=w331, "Cluster"=w283, "error in (no error)"=w330, "Stop Simulation"="StopSim", "filter"="filter") -> ("connection ID out"=w329:refnum<k5>, "Velocity"=w285:cluster{"vx":dbl, "vy":dbl, "vy":dbl}, "Acceleration"=w284:cluster{"ax":dbl, "ay":dbl, "az":dbl}, "Speed"=→"speed":i32, "Simulation Ended"=w327:bool, "error out"=w328:errorcluster)  [unwired: 5 in]
        "acc" <- w284
        "vel" <- w285
        n221 = call "MCA.vi"("Velocity"=w285, "xlp"="xlp", "xhp"="xhp", "Acceleration"=w284, "xrl"="pitchLIM", "yrl"="rollLIM", "zl"="heaveLIM", "ylp"="ylp", "yhp"="yhp", "zhp"="zhp") -> ("Rotations"=w294:cluster{"Pitch":dbl, "Roll":dbl, "yaw ":dbl}, "Heave"=w293:dbl)  [unwired: 4 in]
        "platDisWF" <- w293
        n222 = local read "r"() -> (w303:dbl)
        n223 = local read "R"() -> (w302:dbl)
        n224 = local read "z"() -> (w299:dbl)
        n225 = local read "b"() -> (w300:dbl)
        n226 = local read "a"() -> (w301:dbl)
        n227 = call "Inverse Kinematics.vi"("leg"=w300, "h"=w299, "crank"=w301, "B"=w302, "P"=w303, "Heave"=w293, "R"=w294) -> ("motor"=w277:cluster{dbl, dbl, dbl})  [unwired: 4 in]
        "mPos" <- w277
        n228 = case shown="True" w308 {
          tunnel: w312 -> [_ w357]
          tunnel: w311 -> [_ w356]
          tunnel: [refnum<visa-resource-name> refnum ("VISA resource name out") w355] -> w310
          tunnel: [errorcluster {"status"=FALSE, "code"=0, "source"=""} ("error out") w354] -> w309
          tunnel: w277 -> [_ w345]
          frame False {
          }
          frame True {
            w337 = 10 ("lower limit")
            w338 = 170 ("upper limit")
            w348 = "/"
            n229 = Unbundle(w345) -> (w344:dbl, w343:dbl, w342:dbl)
            n230 = To Long Integer(number=w344) -> (32bit integer=w341:i32)
            n231 = To Long Integer(number=w342) -> (32bit integer=w339:i32)
            n232 = To Long Integer(number=w343) -> (32bit integer=w340:i32)
            n233 = In Range and Coerce(upper limit=w338, x=w341, lower limit=w337) -> (coerced(x)=w336:i32)  [unwired: 1 out]
            n234 = In Range and Coerce(upper limit=w338, x=w340, lower limit=w337) -> (coerced(x)=w335:i32)  [unwired: 1 out]
            n235 = In Range and Coerce(upper limit=w338, x=w339, lower limit=w337) -> (coerced(x)=w334:i32)  [unwired: 1 out]
            n236 = Number To Decimal String(number=w335, width (-)=i16 3) -> (decimal integer string=w349:string)
            n237 = Number To Decimal String(number=w336, width (-)=i16 3) -> (decimal integer string=w350:string)
            n238 = Number To Decimal String(number=w334, width (-)=i16 3) -> (decimal integer string=w347:string)
            n239 = Concatenate Strings(w350, w348, w349, w348, w347) -> (w346:string)
            n240 = VISA Write(VISA resource name=w356, write buffer=w346, error in (no error)=w357) -> (VISA resource name out=w355:refnum<visa-resource-name>, error out=w354:errorcluster)  [unwired: 1 out]
          }
        }
        n241 = expression code="(x/pi)*180.0" "radians to degrees"(w294) -> (w286:cluster{"Pitch":dbl, "Roll":dbl, "yaw ":dbl})
        "platPosWF" <- w286
        n242 = property on="platDisWF" class="WFChart (strict)"("Visible"="dispMCA") -> ()  [unwired: 2 in, 2 out]
        n243 = property on="platPosWF" class="WFChart (strict)"("Visible"="dispMCA") -> ()  [unwired: 2 in, 2 out]
        n244 = property on="acc" class="WFChart (strict)"("Visible"="dispWaveform") -> ()  [unwired: 2 in, 2 out]
        n245 = property on="vel" class="WFChart (strict)"("Visible"="dispWaveform") -> ()  [unwired: 2 in, 2 out]
        n246 = local read "controlON"() -> (w297:bool)
        n247 = Unbundle(w277) -> (w276:dbl, w275:dbl, w274:dbl)
        n248 = Unbundle(w285) -> ("vx"=w289:dbl, "vy"=w288:dbl, "vy"=w287:dbl)
        n249 = Unbundle(w284) -> ("ax"=w292:dbl, "ay"=w291:dbl, "az"=w290:dbl)
        n250 = Unbundle(w286) -> ("Pitch"=w296:dbl, "Roll"=w295:dbl)  [unwired: 1 out]
        n251 = property on="Tab Control 2" class="TabCtl (strict)"("Visible"="Preferences") -> ()  [unwired: 2 in, 2 out]
        n252 = property on="mPos" class="WFChart (strict)"("Visible"=w297) -> ()  [unwired: 2 in, 2 out]
      }
      n253 = property on="Preferences" class="Bool (strict)"("Visible"=TRUE) -> ()  [unwired: 2 in, 2 out]
      n254 = property on="StopSim" class="Bool"("Visible"=TRUE) -> ()  [unwired: 2 in, 2 out]
      n255 = property on="speed" class="Knob (strict)"("Visible"=TRUE) -> ()  [unwired: 2 in, 2 out]
      n256 = local write "Status"("Simulation is Runing" ("String")) -> ()
    }
    frame #4 {
      w437 = TRUE ("Visible")
      # "Post-Simulation"
      n257 = case shown="True" w422 {
        tunnel: w439 -> [_ w480]
        tunnel: w438 -> [_ w479]
        tunnel: [errorcluster {"status"=FALSE, "code"=0, "source"=""} ("error out") w478] -> w424
        frame False {
        }
        frame True {
          n258 = VISA Close(VISA resource name=w480, error in (no error)=w479) -> (error out=w478:errorcluster)
        }
      }
      n259 = local read "record"() -> (w427:bool)
      n260 = TCP Close Connection(connection ID=w421, error in (no error)=w453) -> (error out=w425:errorcluster)  [unwired: 1 in, 1 out]
      n261 = case shown="True" w418 {
        tunnel: w420 -> [_ w456]
        tunnel: w419 -> [_ w455]
        frame False {
        }
        frame True {
          n262 = VISA Close(VISA resource name=w456, error in (no error)=w455) -> ()  [unwired: 1 out]
        }
      }
      n263 = property on="Tab Control 2" class="TabCtl (strict)"("Visible"=FALSE) -> ()  [unwired: 2 in, 2 out]
      n264 = property on="vel" class="WFChart (strict)"("Visible"=TRUE) -> ()  [unwired: 2 in, 2 out]
      n265 = property on="speed" class="Knob (strict)"("Visible"=FALSE) -> ()  [unwired: 2 in, 2 out]
      n266 = property on="acc" class="WFChart (strict)"("Visible"=TRUE) -> ()  [unwired: 2 in, 2 out]
      n267 = property on="StopSim" class="Bool"("Visible"=FALSE) -> ()  [unwired: 2 in, 2 out]
      n268 = property on="Preferences" class="Bool (strict)"("Visible"=FALSE) -> ()  [unwired: 2 in, 2 out]
      n269 = property on="platPosWF" class="WFChart (strict)"("Visible"=TRUE) -> ()  [unwired: 2 in, 2 out]
      n270 = property on="platPosWF" class="WFChart (strict)"("Visible"=FALSE) -> ()  [unwired: 2 in, 2 out]
      n271 = case shown="True" w427 {
        tunnel: w436 -> [_ w476]
        tunnel: w435 -> [_ w475]
        tunnel: w434 -> [_ w474]
        tunnel: w433 -> [_ w473]
        tunnel: w432 -> [_ w472]
        tunnel: w431 -> [_ w471]
        tunnel: w430 -> [_ w470]
        tunnel: w429 -> [_ w469]
        tunnel: w428 -> [_ w468]
        tunnel: [errorcluster {"status"=FALSE, "code"=0, "source"=""} ("error out") w461] -> w426
        tunnel: w417 -> [_ w460]
        tunnel: w416 -> [_ w459]
        tunnel: w415 -> [_ w458]
        frame False {
        }
        frame True {
          n272 = Build Array(w476, w475, w474, w473, w472, w471, w470, w469, w468, w460, w459, w458) -> (w467:dbl[][])
          n273 = local read "report type"() -> (w463:T3)
          n274 = Transpose 2D Array(2D array=w467) -> (transposed array=w464:dbl[][])
          n275 = call <vilib>:"Create Report.vi"("report type"=w463) -> ("report out"=w466:refnum<class "NI_report.lvclass">, "error out"=w465:errorcluster)  [unwired: 13 in]
          n276 = call-poly <vilib>:"Excel Easy Table.vi"("report in"=w466, "text data"=w464, "error in (no error)"=w465, "column headers"=string[] ["Pitch", "Roll", "Heave", "aX", "aY", "aZ", "vX", "vY", "vZ", "m1", "m2", "m3"]) -> ("error out"=w461:errorcluster)  [unwired: 7 in, 4 out]
        }
      }
      n277 = property on="mPos" class="WFChart (strict)"("Visible"=w437) -> ()  [unwired: 2 in, 2 out]
      n278 = property on="platDisWF" class="WFChart (strict)"("Visible"=w437) -> ()  [unwired: 2 in, 2 out]
      n279 = property on="br" class="Knob (strict)"("Visible"=FALSE) -> ()  [unwired: 2 in, 2 out]
      n280 = property on="tr" class="Knob (strict)"("Visible"=FALSE) -> ()  [unwired: 2 in, 2 out]
      n281 = property on="hb" class="Bool (strict)"("Visible"=FALSE) -> ()  [unwired: 2 in, 2 out]
      n282 = property on="rev" class="Bool (strict)"("Visible"=FALSE) -> ()  [unwired: 2 in, 2 out]
      n283 = property on="st" class="Knob (strict)"("Visible"=FALSE) -> ()  [unwired: 2 in, 2 out]
      n284 = Merge Errors(w426, w425, w424) -> (w423:errorcluster)
      n285 = local write "Status"("Simulation has Ended" ("String")) -> ()
      n286 = call <vilib>:"Simple Error Handler.vi"("error in (no error)"=w423) -> ()  [unwired: 4 in, 5 out]
    }
  }
